vi "DG535.constructor.vi"(0 "name":string, 2 "data in":string, 5 "error in(no error)":errorcluster) -> (14 "i ref out":refnum<vi>, 16 "data out":string, 19 "error out":errorcluster)   [LabVIEW 2014, in "DG535.lvlib"]
doc: "Used to control the ds DG535 delay generator.\n\nauthor: R. Savreux, CERN\nmaintainer: R. Savreux, CERN\n\nThis is the constructor of a class.\n\nLicense Agreement for this software:\n\nCopyright (C)\nGesellschaft für Schwerionenforschung, GSI\nPlanckstr. 1\n64291 Darmstadt\nGermany\n\nContact: D.Beck@gsi.de \n\nThis program is free software; you can redistribute it and/or modify it under the terms of the \nGNU General Public License as published by the Free Software Foundation; either version 2 of \nthe license, or (at your option) any later version.\n\nThis program is distributed in the hope that it will be useful, but WITHOUT ANY WARRANTY; \nwithout even the implied warranty of MERCHANTABILITY or FITNESS FOR A PARTICULAR PURPOSE. See the GNU General License for more details (http://www.gnu.org).\n\nGesellschaft für Schwerionenforschung, GSI\nPlanckstr. 1, 64291 Darmstadt, Germany\nFor all questions and ideas contact: M.Richter@gsi.de, H.Brand@gsi.de or D.Beck@gsi.de.\nLast update: 16-JUN-2004"
uses:
  DG535.lvlib
  CSCore/BaseProcess/BaseProcess.lvlib
  CSCore/CSSystem/CSSystemLib/CSSystemLib.lvlib
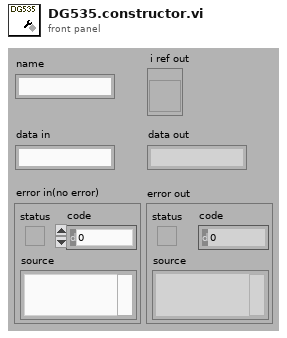
[diagram p1: front panel]
types:
  T1 = enum16{"SetAttribute", "GetAttribute", "CreateAttribute", "DestroyAttribute", "DestroyAllAtributes"}
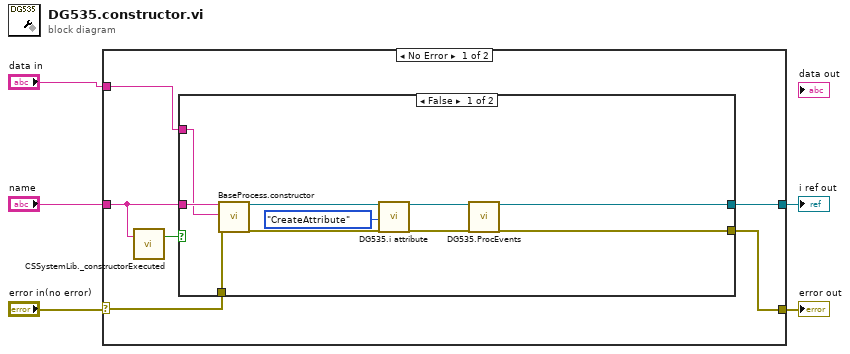
[diagram p0: block diagram]
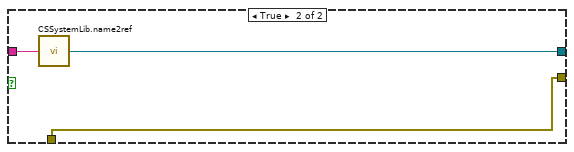
[diagram p2: hidden frame]
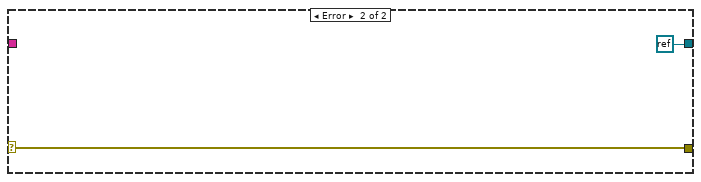
[diagram p3: hidden frame]
diagram:
  n1 = case shown="No Error" "error in(no error)" {
    selector: "error in(no error)" -> [w9 w26]
    tunnel: "name" -> [w7 _]
    tunnel: [w11 refnum<k0> refnum] -> w4
    tunnel: [w10 w26] -> w3
    tunnel: "data in" -> [w6 _]
    frame No Error {
      n2 = call "CSSystemLib._constructorExecuted.vi"("name"=w7) -> ("constructor executed?"=w8:bool)  [unwired: 18 in]
      n3 = case shown="False" w8 {
        tunnel: w7 -> [w18 w23]
        tunnel: [w15 w22] -> w11
        tunnel: [w14 w24] -> w10
        tunnel: w9 -> [w13 w24]
        tunnel: w6 -> [w12 _]
        frame False {
          n4 = call "BaseProcess.constructor.vi"("name"=w18, "data in"=w12, "error in (no error)"=w13) -> ("i ref out"=w21:refnum<vi>, "error out"=w20:errorcluster)  [unwired: 14 in, 1 out]
          n5 = call "DG535.i attribute.vi"("VI Refnum"=w21, "Action"=T1."CreateAttribute", "error in (no error)"=w20) -> ("VI Refnum out"=w17:refnum<vi>, "error out"=w16:errorcluster)  [unwired: 14 in, 1 out]
          n6 = call "DG535.ProcEvents.vi"("i ref in"=w17, "error in"=w16) -> ("i ref out"=w15:refnum<vi>, "error out"=w14:errorcluster)  [unwired: 16 in]
        }
        frame True {
          n7 = call "CSSystemLib.name2ref.vi"("name"=w23) -> ("obj refnum"=w22:refnum<vi>)
        }
      }
    }
    frame Error {
    }
  }
  "i ref out" <- w4
  "error out" <- w3
